vi "XML_GetAncestor.vi"(8 "error in (no error)":errorcluster, 11 "node in":refnum<k20>) -> (0 "error out":errorcluster, 2 "output cluster":T1, 3 "node out":refnum<k20>)   [LabVIEW 2022 SP3, in "ViPER.lvlib" / "ViPER.lvclass"]
uses:
  ViPER.lvclass
  Ancestor.ctl
  <vilib>/xml/Close Reference(Node).vi
  <vilib>/xml/NI_XML.lvlib
  <resource>/objmgr/DOMUserDefRef.rc
panel:
  # "### BSD License (http://www.opensource.org/licenses/bsd-license.php) Begin ###\n\nCopyright (c) 2018  Kurt Friday www.medulla.net\n\nAll rights reserved.\n\nRedistribution and use in source and binary forms, with or without\nmodification, are permitted provided that the following conditions are met:\n\n    * Redistributions of source code must retain the above copyright\n      notice, this list of conditions and the following disclaimer.\n\n    * Redistributions in binary form must reproduce the above copyright\n      notice, this list of conditions and the following disclaimer in the\n      documentation and/or other materials provided with the distribution.\n\n    * Neither the name of the <organization> nor the\n      names of its contributors may be used to endorse or promote products\n      derived from this software without specific prior written permission.\n\nTHIS SOFTWARE IS PROVIDED BY THE COPYRIGHT HOLDERS AND CONTRIBUTORS \"AS IS\" AND\nANY EXPRESS OR IMPLIED WARRANTIES, INCLUDING, BUT NOT LIMITED TO, THE IMPLIED\nWARRANTIES OF MERCHANTABILITY AND FITNESS FOR A PARTICULAR PURPOSE ARE\nDISCLAIMED. IN NO EVENT SHALL <COPYRIGHT HOLDER> BE LIABLE FOR ANY\nDIRECT, INDIRECT, INCIDENTAL, SPECIAL, EXEMPLARY, OR CONSEQUENTIAL DAMAGES\n(INCLUDING, BUT NOT LIMITED TO, PROCUREMENT OF SUBSTITUTE GOODS OR SERVICES;\nLOSS OF USE, DATA, OR PROFITS; OR BUSINESS INTERRUPTION) HOWEVER CAUSED AND\nON ANY THEORY OF LIABILITY, WHETHER IN CONTRACT, STRICT LIABILITY, OR TORT\n(INCLUDING NEGLIGENCE OR OTHERWISE) ARISING IN ANY WAY OUT OF THE USE OF THIS\nSOFTWARE, EVEN IF ADVISED OF THE POSSIBILITY OF SUCH DAMAGE."
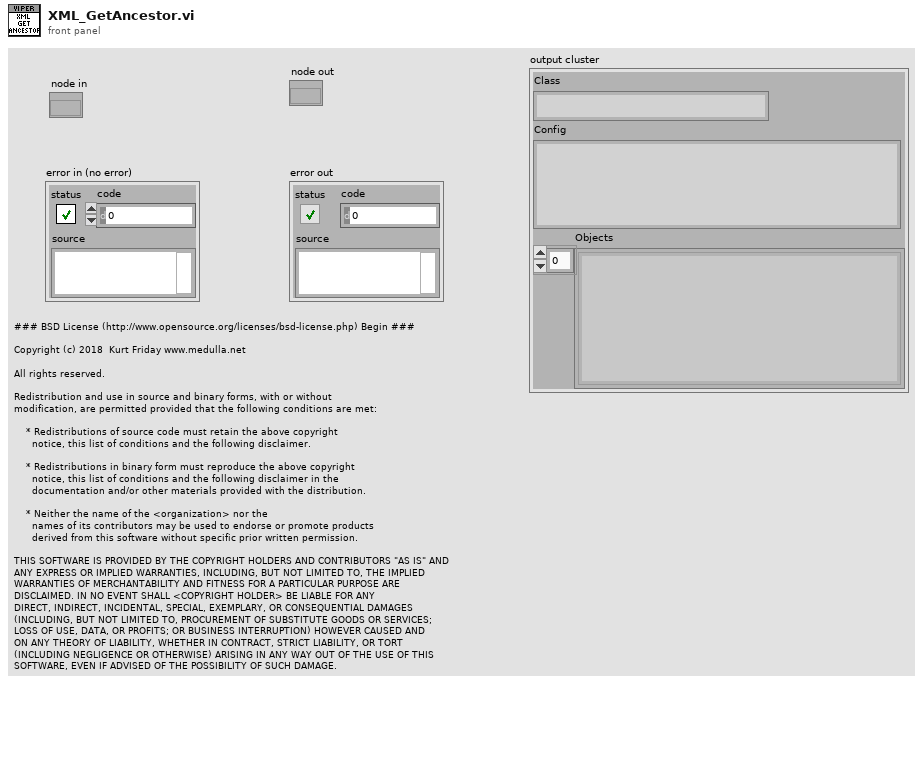
[diagram p1: front panel]
types:
  T1 = typedef "ViPER.lvlib/ViPER.lvclass/Ancestor.ctl" = cluster{"Class":string, "Config":string, "Objects":string[]}
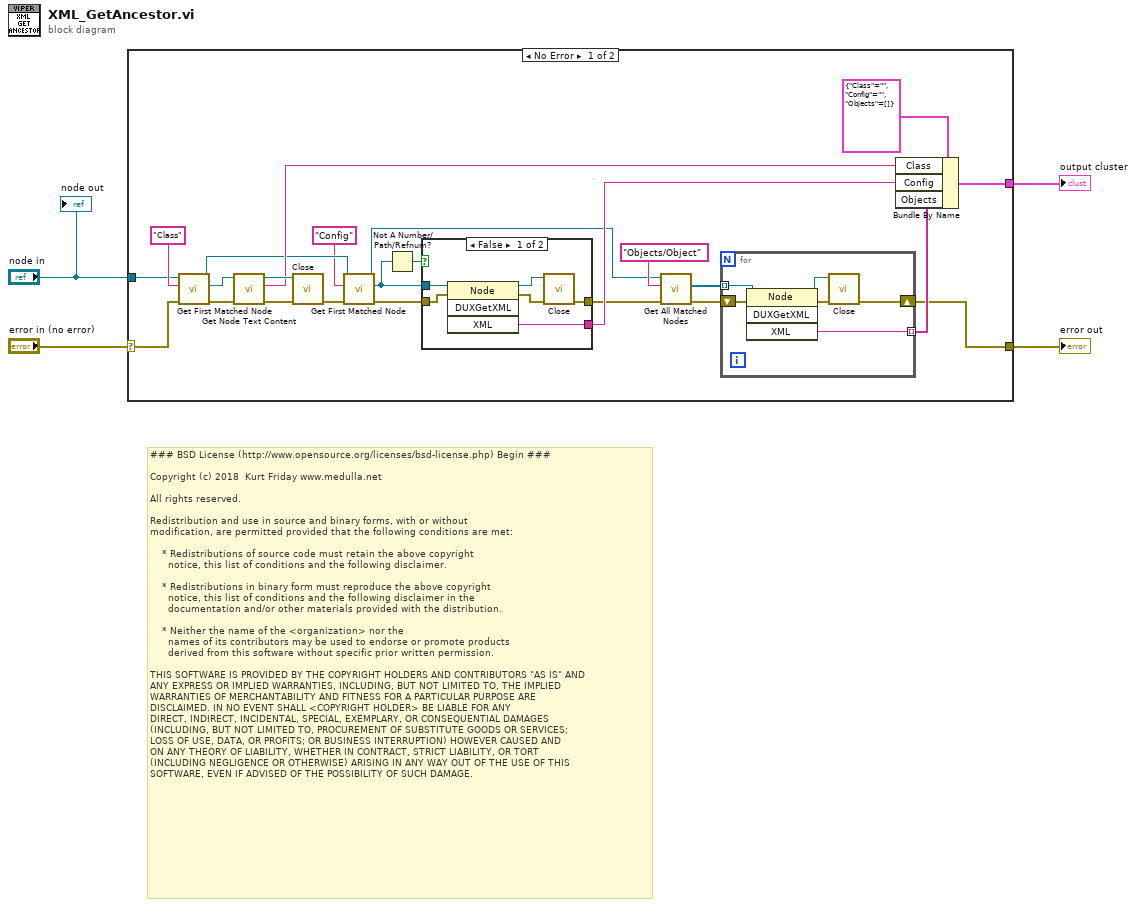
[diagram p0: block diagram]
diagram:
  # "### BSD License (http://www.opensource.org/licenses/bsd-license.php) Begin ###\n\nCopyright (c) 2018  Kurt Friday www.medulla.net\n\nAll rights reserved.\n\nRedistribution and use in source and binary forms, with or without\nmodification, are permitted provided that the following conditions are met:\n\n    * Redistributions of source code must retain the above copyright\n      notice, this list of conditions and the following disclaimer.\n\n    * Redistributions in binary form must reproduce the above copyright\n      notice, this list of conditions and the following disclaimer in the\n      documentation and/or other materials provided with the distribution.\n\n    * Neither the name of the <organization> nor the\n      names of its contributors may be used to endorse or promote products\n      derived from this software without specific prior written permission.\n\nTHIS SOFTWARE IS PROVIDED BY THE COPYRIGHT HOLDERS AND CONTRIBUTORS \"AS IS\" AND\nANY EXPRESS OR IMPLIED WARRANTIES, INCLUDING, BUT NOT LIMITED TO, THE IMPLIED\nWARRANTIES OF MERCHANTABILITY AND FITNESS FOR A PARTICULAR PURPOSE ARE\nDISCLAIMED. IN NO EVENT SHALL <COPYRIGHT HOLDER> BE LIABLE FOR ANY\nDIRECT, INDIRECT, INCIDENTAL, SPECIAL, EXEMPLARY, OR CONSEQUENTIAL DAMAGES\n(INCLUDING, BUT NOT LIMITED TO, PROCUREMENT OF SUBSTITUTE GOODS OR SERVICES;\nLOSS OF USE, DATA, OR PROFITS; OR BUSINESS INTERRUPTION) HOWEVER CAUSED AND\nON ANY THEORY OF LIABILITY, WHETHER IN CONTRACT, STRICT LIABILITY, OR TORT\n(INCLUDING NEGLIGENCE OR OTHERWISE) ARISING IN ANY WAY OUT OF THE USE OF THIS\nSOFTWARE, EVEN IF ADVISED OF THE POSSIBILITY OF SUCH DAMAGE."
  n1 = case shown="No Error" "error in (no error)" {
    selector: "error in (no error)" -> [w5 w42]
    tunnel: "node in" -> [w8 _]
    tunnel: [w7 w42] -> w3
    tunnel: [w6 _] -> w2
    frame No Error {
      n2 = call <vilib>:"Get First Matched Node.vi"("error in (no error)"=w5, "XPath expression"="Class", "node in"=w8) -> ("error out"=w27:errorcluster, "node result"=w26:refnum<k20>, "node out"=w20:refnum<k20>)  [unwired: 6 in]
      n3 = call <vilib>:"Get Node Text Content.vi"("error in (no error)"=w27, "node in"=w26) -> ("error out"=w25:errorcluster, "node text"=w22:string, "node out"=w24:refnum<k20>)  [unwired: 7 in]
      n4 = call-poly <vilib>:"Close.vi"("error in (no error)"=w25, "node"=w24) -> ("error out"=w21:errorcluster)  [unwired: 7 out]
      n5 = call <vilib>:"Get First Matched Node.vi"("error in (no error)"=w21, "XPath expression"="Config", "node in"=w20) -> ("error out"=w17:errorcluster, "node result"=w18:refnum<k20>, "node out"=w10:refnum<k20>)  [unwired: 6 in]
      n6 = Not A Number/Path/Refnum?(number/path/refnum=w18) -> (NaN/Path/Refnum?=w19:bool)
      n7 = case shown="False" w19 {
        tunnel: w18 -> [w40 _]
        tunnel: w17 -> [w39 w41]
        tunnel: [w36 w41] -> w15
        tunnel: [w38 _] -> w16
        frame False {
          n8 = invoke on="Invoke Node" class="Node" method="DUXGetXML"(reference=w40, error in=w39) -> (reference out=w35:refnum<k20>, error out=w37:errorcluster, "XML"=w38:string)  [unwired: 2 in, 1 out]
          n9 = call-poly <vilib>:"Close.vi"("error in (no error)"=w37, "node"=w35) -> ("error out"=w36:errorcluster)  [unwired: 7 out]
        }
        frame True {
        }
      }
      n10 = call <vilib>:"Get All Matched Nodes.vi"("error in (no error)"=w15, "XPath expression"="Objects/Object", "node in"=w10) -> ("error out"=w12:errorcluster, "node result array"=w11:refnum<k20>[])  [unwired: 6 in, 1 out]
      n11 = for {
        tunnel: w11 -> [w34] mode=indexing
        shift-right: [w30] -> w7
        shift-left: w12 -> [w33]
        tunnel: [w32] -> w9 mode=indexing
        n12 = invoke on="Invoke Node" class="Node" method="DUXGetXML"(reference=w34, error in=w33) -> (reference out=w29:refnum<k20>, error out=w31:errorcluster, "XML"=w32:string)  [unwired: 2 in, 1 out]
        n13 = call-poly <vilib>:"Close.vi"("error in (no error)"=w31, "node"=w29) -> ("error out"=w30:errorcluster)  [unwired: 7 out]
      }
      n14 = Bundle By Name(cluster=T1 {"Class"="", "Config"="", "Objects"=[]} ("Layer"), "Class"=w22, "Config"=w16, "Objects"=w9) -> (w6:T1)
    }
    frame Error {
    }
  }
  "error out" <- w3
  "output cluster" <- w2
  "node out" <- "node in"
